vi "Write Wash Step Indicators.vi"(8 "error in (no error)":errorcluster, 10 "Wash Step Indicators":refnum<vi>, 11 "Wash Display Console in":refnum<class "Wash Display Console.lvclass">) -> (0 "error out":errorcluster, 3 "Wash Display Console out":refnum<class "Wash Display Console.lvclass">)   [LabVIEW 2013, in "Wash Display Console.lvlib" / "Wash Display Console.lvclass"]
uses:
  Wash Display Console.lvclass
  Wash Display Console.lvclass/Wash Display Console.ctl
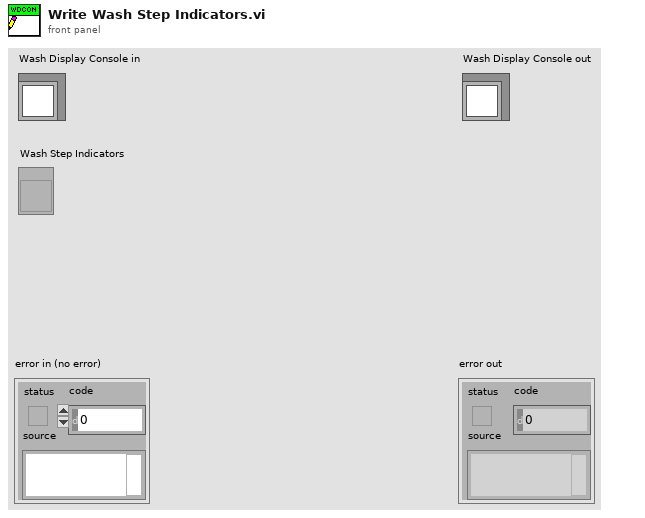
[diagram p1: front panel]
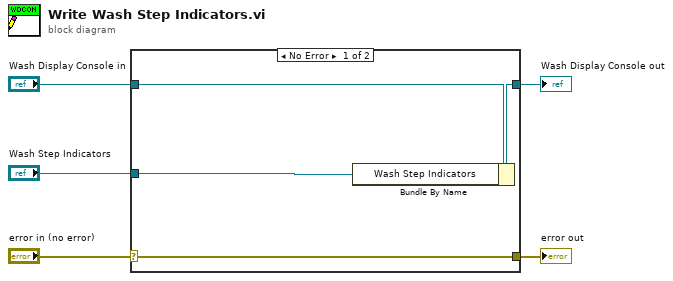
[diagram p0: block diagram]
diagram:
  n1 = case shown="No Error" "error in (no error)" {
    selector: "error in (no error)" -> [w9 w10]
    tunnel: [w9 w10] -> w4
    tunnel: [w7 w11] -> w2
    tunnel: "Wash Display Console in" -> [w8 w11]
    tunnel: "Wash Step Indicators" -> [w6 _]
    frame No Error {
      n2 = Bundle By Name(cluster=w8, "Wash Step Indicators"=w6) -> (w7:refnum<class "Wash Display Console.lvclass">)
    }
    frame Error {
    }
  }
  "error out" <- w4
  "Wash Display Console out" <- w2
